vi "Read Rect.vi"(11 "Rectangle in":refnum<class "Rectangle.lvclass">) -> (2 "rect":T1)   [LabVIEW 2024, in "Rectangle.lvclass"]
doc: "MIT Licence\nCopyright (c) 2024 David Grollier"
uses:
  Rectangle.lvclass
  Rectangle.lvclass/Rectangle.ctl
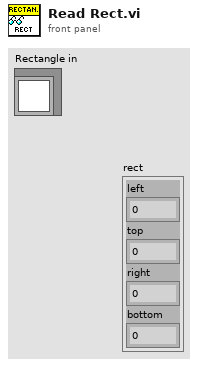
[diagram p1: front panel]
types:
  T1 = cluster{"left":i16, "top":i16, "right":i16, "bottom":i16}
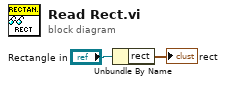
[diagram p0: block diagram]
diagram:
  n1 = Unbundle By Name("Rectangle in") -> ("rect"=→"rect":T1)
